vi "AOL Z Cal load-Bring to front.vi"   [LabVIEW 2020]
uses:
  Configuration code/Calibration/Globals/gl_Calibration globals.vi
types:
  T1 = enum32{"Invalid", "Standard", "Closed", "Hidden", "Minimized", "Maximized"}
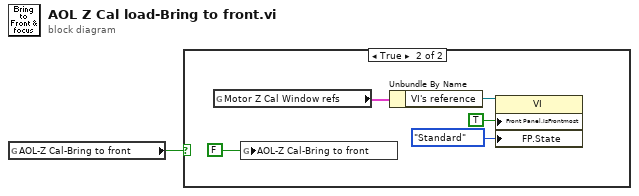
[diagram p0: block diagram]
diagram:
  n1 = global read "gl_Calibration globals.vi" "AOL-Z Cal-Bring to front"() -> (w1:bool)
  n2 = case shown="True" w1 {
    frame False {
    }
    frame True {
      n3 = global read "gl_Calibration globals.vi" "Motor Z Cal Window refs"() -> (w2:cluster{"VI's reference":refnum<vi>})
      n4 = global write "gl_Calibration globals.vi" "AOL-Z Cal-Bring to front"(FALSE ("Bring to front")) -> ()
      n5 = Unbundle By Name(w2) -> ("VI's reference"=w4:refnum<vi>)
      n6 = property class="VI"(reference=w4, "Front Panel.IsFrontmost"=TRUE ("Front Panel Window:Is Frontmost"), "FP.State"=T1."Standard" ("Front Panel Window:State")) -> ()  [unwired: 1 in, 2 out]
    }
  }
